vi "Example.vi"() -> ()   [LabVIEW 2018]
uses:
  <userlib>/DAQNavi Polymorphic VI/create/DAQNavi Create Channel(AI-Voltage).vi
  <userlib>/DAQNavi Polymorphic VI/configure/timing/DAQNavi Timing(AI Convert Clock).vi
  <userlib>/DAQNavi Polymorphic VI/read/DAQNavi Read (Analog 1D Wfm NChan NSamp).vi
  <userlib>/DAQNavi Polymorphic VI/configure/DAQNavi Get Property/Device/DAQNaviGet_Device_SupportedDevices_Ex.vi
  <vilib>/gmath/NI_Gmath.lvlib
panel:
  in  "MeanType":T1(ring)
  in  "Settings":T2(array[cluster])
  in  "Refresh Button":bool
  out "Acture Storage Period (s)":dbl=0.1 caption="Acture" min=0.001 format="%#_6p"
  out "Acture Refresh Period (s)":dbl=0.1 caption="Acture" min=0.001 format="%#_6p"
  in  "Storage Period (s)":dbl=0.1 min=0.001 format="%#_6p"
  out "File Path":path
  out "Recording":bool
  out "Over\nrun?":bool
  in  "Record Button":bool
  in  "Refresh Period (s)":dbl=0.1 min=0.001 format="%#_6p"
  in  "Process Stop Button":bool
  in  "Stop Button":bool
  in  "Play Button":bool
  out "Waveform Chart":waveform(dbl)[](graph)
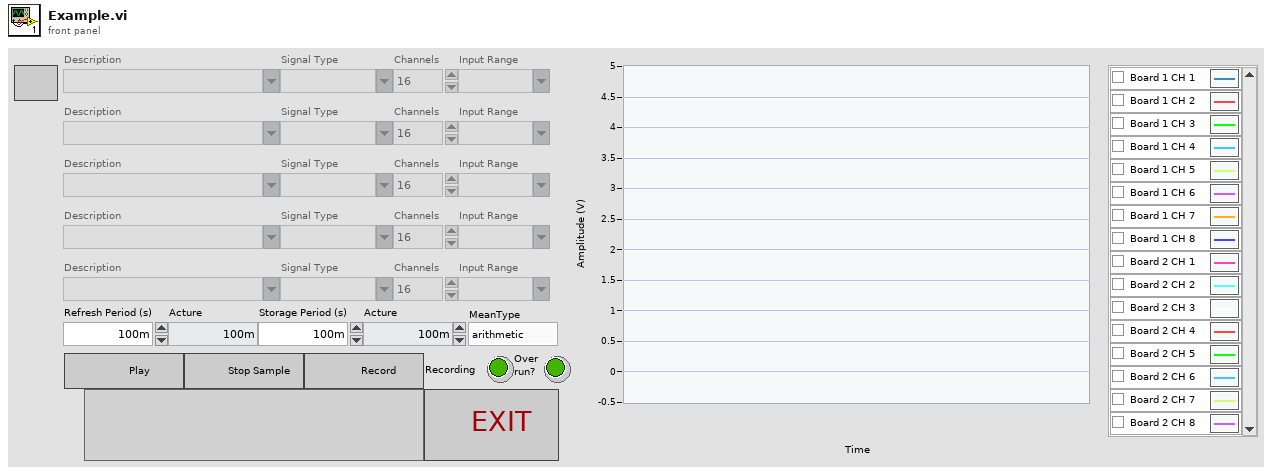
[diagram p1: front panel]
types:
  T1 = enum16{"arithmetic", "geometric", "harmonic", "trimmed", "median"}
  T2 = cluster{"Description":string, "Signal Type":string, "Channels":i32, "Input Range":string}[]
  T3 = enum16{"Close and Open", "Write", "Write Header", "Close"}
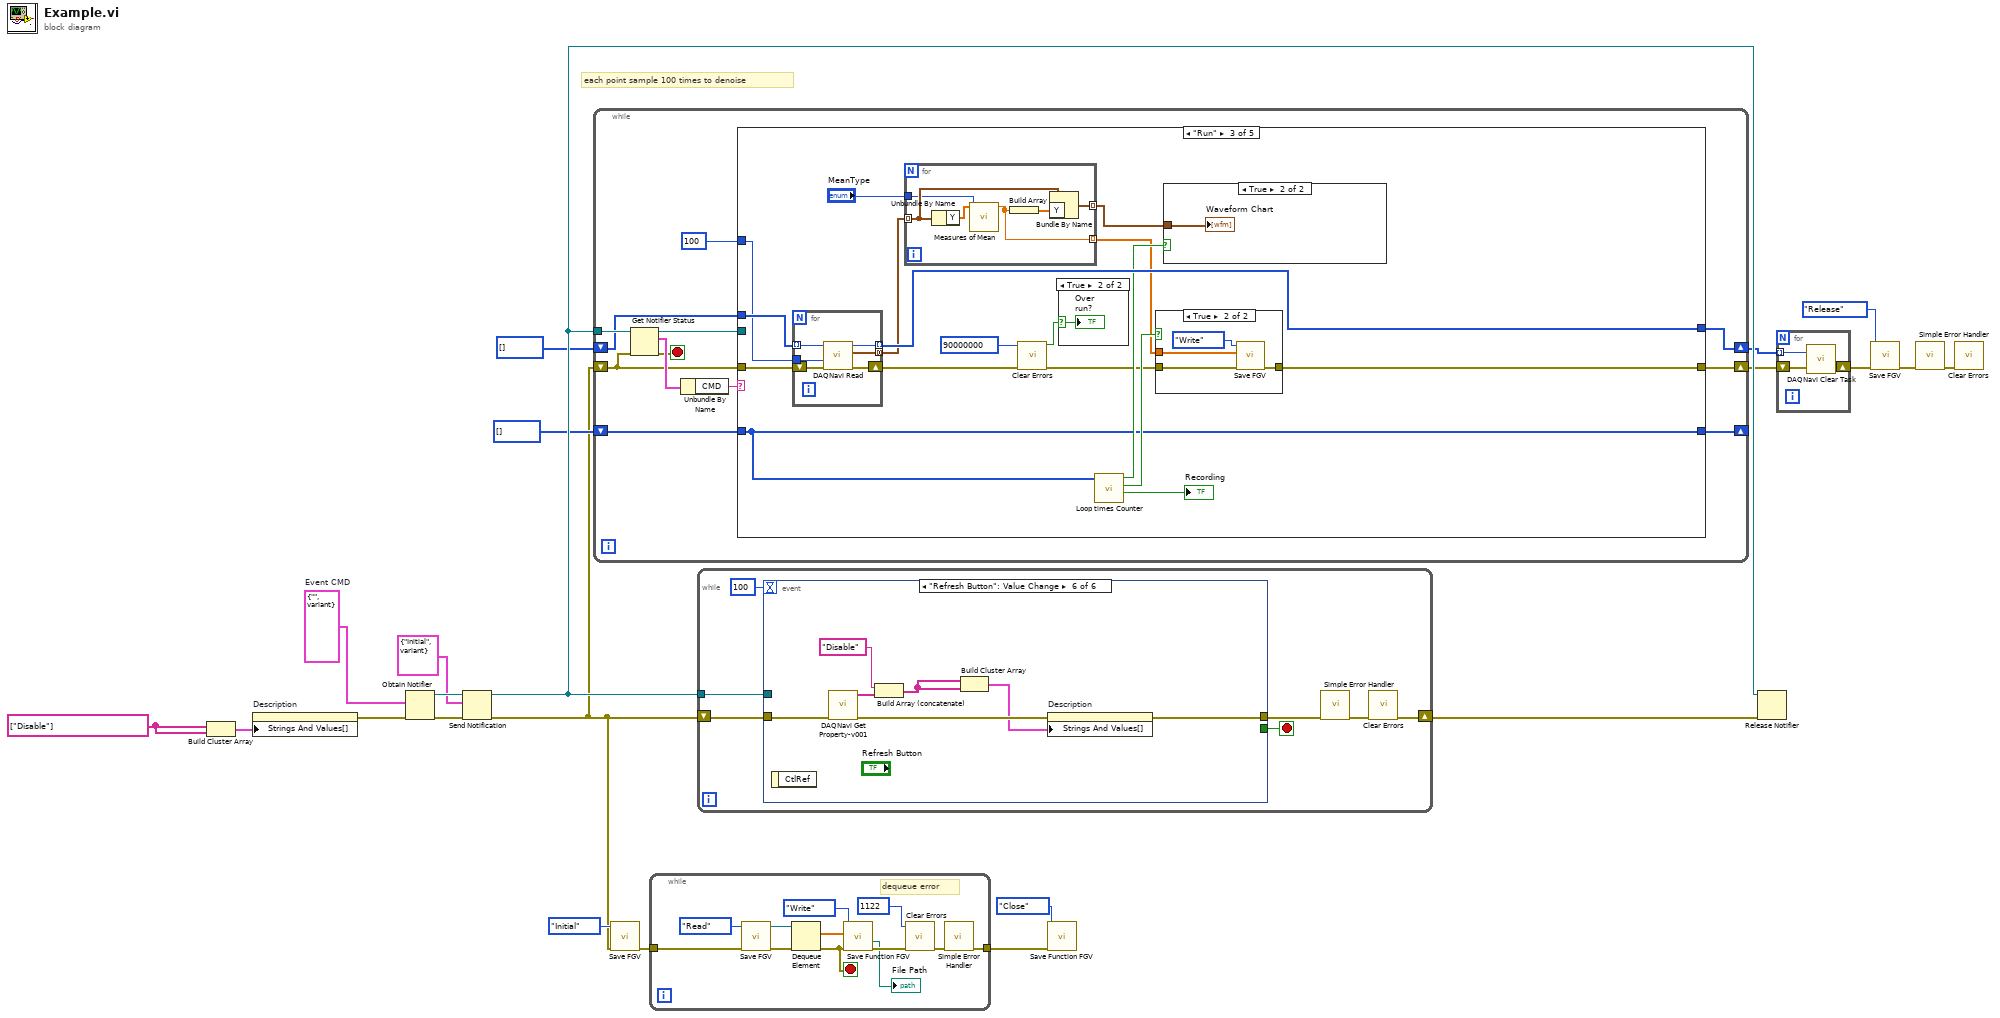
[diagram p0: block diagram]
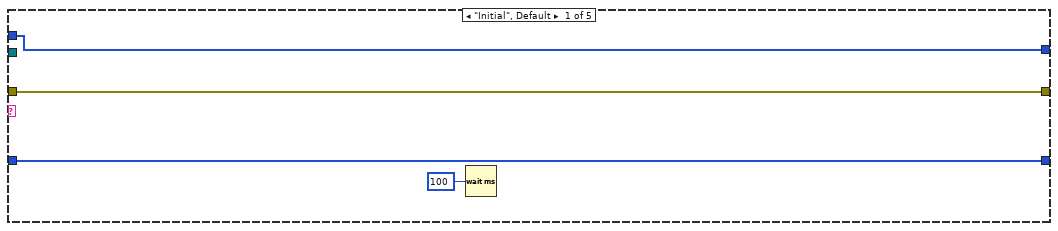
[diagram p2: hidden frame]
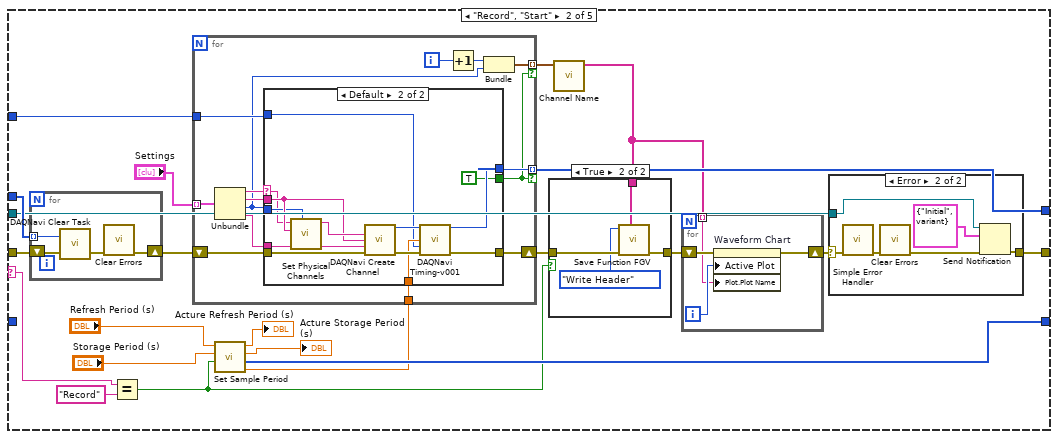
[diagram p3: hidden frame]
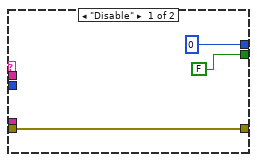
[diagram p5: hidden frame]
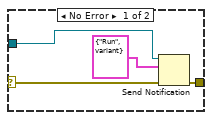
[diagram p6: hidden frame]
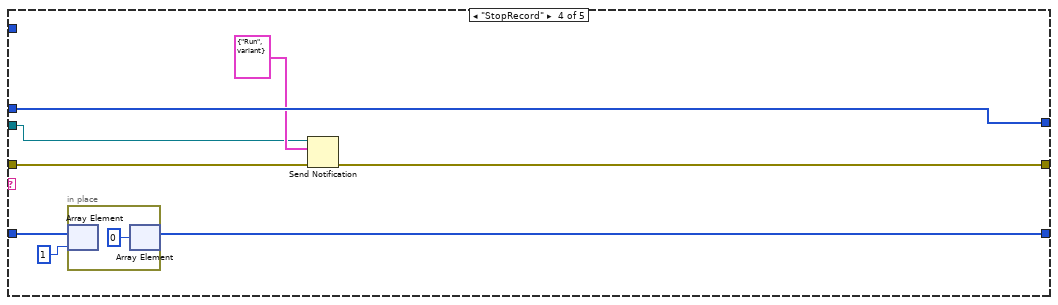
[diagram p10: hidden frame]
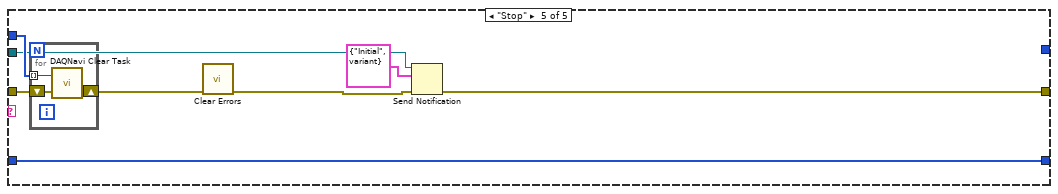
[diagram p11: hidden frame]
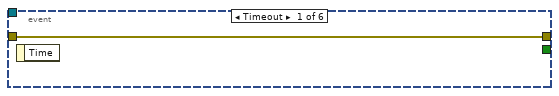
[diagram p12: hidden frame]
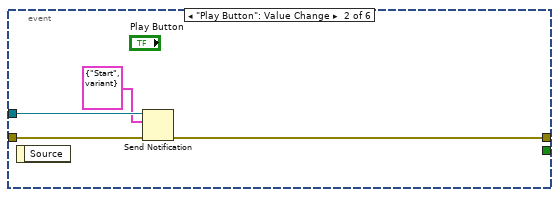
[diagram p13: hidden frame]
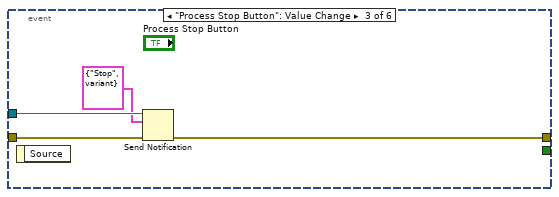
[diagram p14: hidden frame]
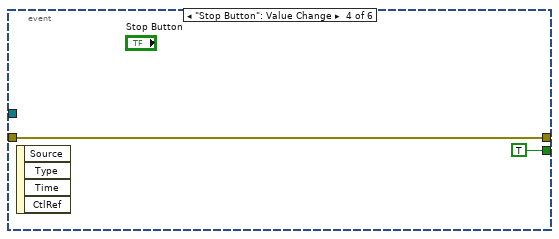
[diagram p15: hidden frame]
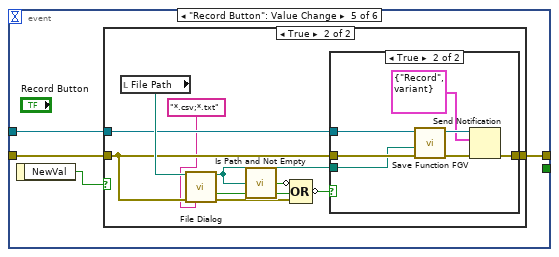
[diagram p16: hidden frame]
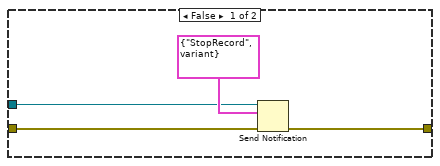
[diagram p17: hidden frame]
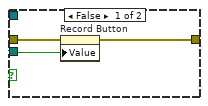
[diagram p18: hidden frame]
diagram:
  w3 = string[] ["Disable"]
  w22 = cluster{"CMD":string, "Data":variant} {"CMD"="", "Data"=variant}  # Event CMD
  # "each point sample 100 times to denoise"
  n1 = Build Cluster Array(w3, w3) -> (w2:cluster{"String":string, "String":string}[])
  n2 = property on="Description" class="CmbBox"("Strings And Values[]"=w2) -> (error out=w1:errorcluster)  [unwired: 2 in, 1 out]
  n3 = Obtain Notifier(notification data type=w22, error in (no error)=w1) -> (notifier out=w21:refnum<notifier>, error out=w19:errorcluster)  [unwired: 2 in, 1 out]
  n4 = Send Notification(notification=cluster{"CMD":string, "Data":variant} {"CMD"="Initial", "Data"=variant} ("element"), notifier=w21, error in (no error)=w19) -> (notifier out=w17:refnum<notifier>, error out=w10:errorcluster)
  n5 = while {
    tunnel: w17 -> [w34]
    shift-right: [w29] -> w7
    shift-left: i32[] [] ("task out") -> [w28]
    shift-right: [w24] -> w6
    shift-left: w10 -> [w30]
    shift-right: [w26] -> _
    shift-left: i32[] [] ("times") -> [w25]
    stop <- w31 stop-if-true
    n6 = Get Notifier Status(notifier=w34, error in (no error)=w30) -> (notifier out=w27:refnum<notifier>, current notification=w33:cluster{"CMD":string, "Data":variant}, error out=w31:errorcluster)  [unwired: 2 out]
    n7 = Unbundle By Name(w33) -> ("CMD"=w32:string)
    n8 = case shown="\"Run\"" w32 {
      selector: w32 -> [_ w45 _ _ _]
      tunnel: w30 -> [w38 w59 w125 w152 w164]
      tunnel: [w38 w51 w119 w151 w162] -> w24
      tunnel: [w37 w50 w129 w157 _] -> w29
      tunnel: w28 -> [w37 w60 w130 w157 w165]
      tunnel: w27 -> [_ w57 _ w150 w161]
      tunnel: [w35 w52 w122 w154 w159] -> w26
      tunnel: w25 -> [w35 _ w122 w156 w159]
      tunnel: u32 100 ("section length") -> [_ w48 w118 _ _]
      frame "Initial", Default {
        n9 = Wait (ms)(milliseconds to wait=u32 100) -> ()  [unwired: 1 out]
      }
      frame "Record", "Start" {
        n10 = for {
          tunnel: w60 -> [w73] mode=indexing
          shift-right: [w70] -> w58
          shift-left: w59 -> [w71]
          n11 = call <userlib>:"DAQNavi Clear Task.vi"("error in (no error)"=w71, "task in"=w73) -> ("error out"=w72:errorcluster)  [unwired: 1 out]
          n12 = call <vilib>:"Clear Errors.vi"("error in (no error)"=w72) -> ("error out"=w70:errorcluster)  [unwired: 5 in, 1 out]
        }
        n13 = Equal?(x=w45, y="Record") -> (x = y?=w43:bool)
        n14 = call "Set Sample Period.vi"("Record?"=w43, "Storage Period (s)"="Storage Period (s)", "Refresh Period (s)"="Refresh Period (s)") -> ("Rate"=w49:dbl, "times"=w52:i32[], "Acture Storage Period (s)"=→"Acture Storage Period (s)":dbl, "Acture Refresh Period (s)"=→"Acture Refresh Period (s)":dbl)  [unwired: 5 in]
        n15 = for {
          tunnel: [w85] -> w50 mode=indexing if=w74
          tunnel: w49 -> [w84]
          tunnel: w48 -> [w83]
          shift-right: [w86] -> w44
          shift-left: w58 -> [w87]
          tunnel: "Settings" -> [w82] mode=indexing
          tunnel: [w75] -> w42 mode=indexing if=w74
          i -> [w78]
          n16 = Unbundle(w82) -> ("Description"=w79:string, "Signal Type"=w81:string, "Channels"=w76:i32, "Input Range"=w80:string)
          n17 = case shown="Default" w79 {
            selector: w79 -> [_ w92]
            tunnel: w80 -> [_ w102]
            tunnel: w87 -> [w89 w101]
            tunnel: [w89 w98] -> w86
            tunnel: [0 ("task out") w97] -> w85
            tunnel: w84 -> [_ w96]
            tunnel: w83 -> [_ w95]
            tunnel: w81 -> [_ w94]
            tunnel: w76 -> [_ w93]
            tunnel: [FALSE TRUE] -> w74
            frame "Disable" {
            }
            frame Default {
              n18 = call "Set Physical Channels.vi"("Channels"=w93, "signal type"=w94, "Board Description"=w92) -> ("String"=w103:string)  [unwired: 8 in]
              n19 = call-poly <userlib>:"DAQNavi Create Channel.vi"("physical channels"=w103, "signal type"=w94, "value range"=w102, "error in (no error)"=w101) -> ("task out"=w100:i32, "error out"=w99:errorcluster)  [unwired: 1 in, 9 out]
              n20 = call-poly <userlib>:"DAQNavi Timing-v001.vi"("task in"=w100, "rate"=w96, "section length"=w95, "error in (no error)"=w99) -> ("task out"=w97:i32, "error out"=w98:errorcluster)  [unwired: 3 in, 7 out]
            }
          }
          n21 = Increment(x=w78) -> (x+1=w77:i32)
          n22 = Bundle(w77, "Channels"=w76) -> (w75:cluster{i32, "Channels":i32})  [unwired: 1 in]
        }
        n23 = call "Channel Name.vi"("Channel property"=w42) -> ("Channel Name"=w39:string[])  [unwired: 10 in]
        n24 = case shown="True" w43 {
          tunnel: w44 -> [w65 w69]
          tunnel: [w65 w68] -> w41
          tunnel: w39 -> [_ w67]
          frame False {
          }
          frame True {
            n25 = call "Save Function FGV.vi"("Channel Name in"=w67, "error in"=w69, "CMD"=T3."Write Header") -> ("error out"=w68:errorcluster)  [unwired: 6 in, 2 out]
          }
        }
        n26 = for {
          shift-right: [w63] -> w40
          shift-left: w41 -> [w64]
          tunnel: w39 -> [w61] mode=indexing
          i -> [w62]
          n27 = property on="Waveform Chart" class="WFChart (strict)"(error in=w64, "Active Plot"=w62, "Plot.Plot Name"=w61) -> (error out=w63:errorcluster)  [unwired: 1 in, 1 out]
        }
        n28 = case shown="Error" w40 {
          selector: w40 -> [w104 w110]
          tunnel: w57 -> [w107 w112]
          tunnel: [w106 w111] -> w51
          frame No Error {
            n29 = Send Notification(notification=cluster{"CMD":string, "Data":variant} {"CMD"="Run", "Data"=variant} ("element"), notifier=w107, error in (no error)=w104) -> (error out=w106:errorcluster)  [unwired: 1 out]
          }
          frame Error {
            n30 = call <vilib>:"Simple Error Handler.vi"("error in (no error)"=w110) -> ("error out"=w109:errorcluster)  [unwired: 4 in, 4 out]
            n31 = call <vilib>:"Clear Errors.vi"("error in (no error)"=w109) -> ("error out"=w108:errorcluster)  [unwired: 5 in, 1 out]
            n32 = Send Notification(notification=cluster{"CMD":string, "Data":variant} {"CMD"="Initial", "Data"=variant} ("element"), notifier=w112, error in (no error)=w108) -> (error out=w111:errorcluster)  [unwired: 1 out]
          }
        }
      }
      frame "Run" {
        n33 = for {
          tunnel: w130 -> [w136] mode=indexing
          tunnel: [w135] -> w129 mode=indexing
          tunnel: w118 -> [w132]
          tunnel: [w131] -> w116 mode=concatenating
          shift-right: [w134] -> w128
          shift-left: w125 -> [w133]
          n34 = call-poly <userlib>:"DAQNavi Read.vi"("error in (no error)"=w133, "number of samples per channel to read"=w132, "task in"=w136) -> ("error out"=w134:errorcluster, "data"=w131:waveform(dbl)[], "task out"=w135:i32)  [unwired: 1 in, 5 out]
        }
        n35 = for {
          tunnel: w116 -> [w145] mode=indexing
          tunnel: [w146] -> w115 mode=indexing
          tunnel: [w148] -> w117 mode=indexing
          tunnel: "MeanType" -> [w144]
          n36 = Unbundle By Name(w145) -> ("Y"=w149:dbl[])
          n37 = call <vilib>:"Measures of Mean.vi"("type"=w144, "x array"=w149) -> ("mean value"=w148:dbl)  [unwired: 8 in, 1 out]
          n38 = Build Array(w148) -> (w147:dbl[])
          n39 = Bundle By Name(cluster=w145, "Y"=w147) -> (w146:waveform(dbl))
        }
        n40 = call <vilib>:"Clear Errors.vi"("error in (no error)"=w128, "specific error code to clear (0: all)"=90000000) -> ("error out"=w120:errorcluster, "specific error cleared?"=w126:bool)  [unwired: 4 in]
        n41 = case shown="True" w126 {
          selector: w126 -> [_ w143]
          frame False {
          }
          frame True {
            "Over\nrun?" <- w143
          }
        }
        n42 = call "Loop times Counter.vi"("times"=w122) -> ("Recording?"=→"Recording":bool, "Save file?"=w123:bool, "Display value?"=w124:bool)  [unwired: 8 in]
        n43 = case shown="True" w123 {
          tunnel: w117 -> [_ w141]
          tunnel: w120 -> [w137 w140]
          tunnel: [w137 w138] -> w119
          frame False {
          }
          frame True {
            n44 = call "Save FGV.vi"("error in (no error)"=w140, "Data in"=w141, "CMD"=enum16{"Initial", "Read", "Write", "Release"}."Write") -> ("error out"=w138:errorcluster)  [unwired: 7 in, 1 out]
          }
        }
        n45 = case shown="True" w124 {
          tunnel: w115 -> [_ w142]
          frame False {
          }
          frame True {
            "Waveform Chart" <- w142
          }
        }
      }
      frame "StopRecord" {
        n46 = in-place {
          n47 = in-place-array #1(w156, 1) -> ()  [unwired: 1 out]
          n48 = in-place-array #1(0 ("element")) -> (w154:i32[])  [unwired: 1 out]
        }
        n49 = Send Notification(notification=cluster{"CMD":string, "Data":variant} {"CMD"="Run", "Data"=variant} ("element"), notifier=w150, error in (no error)=w152) -> (error out=w151:errorcluster)  [unwired: 1 out]
      }
      frame "Stop" {
        n50 = for {
          tunnel: w165 -> [w168] mode=indexing
          shift-right: [w169] -> w166
          shift-left: w164 -> [w167]
          n51 = call <userlib>:"DAQNavi Clear Task.vi"("error in (no error)"=w167, "task in"=w168) -> ("error out"=w169:errorcluster)  [unwired: 1 out]
        }
        n52 = call <vilib>:"Clear Errors.vi"("error in (no error)"=w166) -> ("error out"=w163:errorcluster)  [unwired: 5 in, 1 out]
        n53 = Send Notification(notification=cluster{"CMD":string, "Data":variant} {"CMD"="Initial", "Data"=variant} ("element"), notifier=w161, error in (no error)=w163) -> (error out=w162:errorcluster)  [unwired: 1 out]
      }
    }
  }
  n54 = call "Save FGV.vi"("error in (no error)"=w10, "CMD"=enum16{"Initial", "Read", "Write", "Release"}."Initial") -> ("error out"=w12:errorcluster)  [unwired: 8 in, 1 out]
  n55 = while {
    tunnel: w12 -> [w180]
    tunnel: [w173] -> w11
    stop <- w176 stop-if-true
    # "dequeue error"
    n56 = call "Save FGV.vi"("error in (no error)"=w180, "CMD"=enum16{"Initial", "Read", "Write", "Release"}."Read") -> ("error out"=w177:errorcluster, "file queue out"=w179:refnum<queue>)  [unwired: 8 in]
    n57 = Dequeue Element(queue=w179, error in (no error)=w177) -> (element=w178:dbl[], error out=w176:errorcluster)  [unwired: 1 in, 2 out]
    n58 = call "Save Function FGV.vi"("error in"=w176, "data in"=w178, "CMD"=T3."Write") -> ("error out"=w175:errorcluster, "file path out"=→"File Path":path)  [unwired: 6 in, 1 out]
    n59 = call <vilib>:"Clear Errors.vi"("error in (no error)"=w175, "specific error code to clear (0: all)"=1122) -> ("error out"=w174:errorcluster)  [unwired: 4 in, 1 out]
    n60 = call <vilib>:"Simple Error Handler.vi"("error in (no error)"=w174) -> ("error out"=w173:errorcluster)  [unwired: 4 in, 4 out]
  }
  n61 = while {
    tunnel: w17 -> [w188]
    shift-right: [w183] -> w18
    shift-left: w10 -> [w185]
    stop <- w186 stop-if-true
    n62 = event shown="[5] \"Refresh Button\": Value Change" {
      selector: _ -> [_ _ _ _ _ _]
      dyn-events: _ -> [_ _ _ _ _ _]
      timeout: 100 -> [_ _ _ _ _ _]
      tunnel: w188 -> [_ w193 w197 _ w201 _]
      tunnel: [w189 w192 w196 w198 w202 w229] -> w187
      tunnel: [_ _ _ TRUE _ _] -> w186
      tunnel: w185 -> [w189 w190 w194 w198 w203 w233]
      event Timeout {
        n63 = event-data() -> ()  [unwired: 1 in, 1 out]
      }
      event "Play Button": Value Change {
        n64 = event-data() -> ()  [unwired: 1 in, 1 out]
        n65 = Send Notification(notification=cluster{"CMD":string, "Data":variant} {"CMD"="Start", "Data"=variant} ("element"), notifier=w193, error in (no error)=w190) -> (error out=w192:errorcluster)  [unwired: 1 out]
      }
      event "Process Stop Button": Value Change {
        n66 = event-data() -> ()  [unwired: 1 in, 1 out]
        n67 = Send Notification(notification=cluster{"CMD":string, "Data":variant} {"CMD"="Stop", "Data"=variant} ("element"), notifier=w197, error in (no error)=w194) -> (error out=w196:errorcluster)  [unwired: 1 out]
      }
      event "Stop Button": Value Change {
        n68 = event-data() -> ()  [unwired: 1 in, 4 out]
      }
      event "Record Button": Value Change {
        n69 = event-data() -> ("NewVal"=w200:bool)  [unwired: 1 in]
        n70 = case shown="True" w200 {
          tunnel: w203 -> [w205 w211]
          tunnel: [w204 w210] -> w202
          tunnel: w201 -> [w206 w209]
          frame False {
            n71 = Send Notification(notification=cluster{"CMD":string, "Data":variant} {"CMD"="StopRecord", "Data"=variant} ("element"), notifier=w206, error in (no error)=w205) -> (error out=w204:errorcluster)  [unwired: 1 out]
          }
          frame True {
            n72 = local read "File Path"() -> (w212:path)
            n73 = call "File Dialog"("start path"=w212, "error in"=w211, "pattern (all files)"="*.csv;*.txt") -> ("selected path"=w214:path, "cancelled"=w216:bool, "error out"=w215:errorcluster)  [unwired: 9 in, 1 out]
            n74 = call <vilib>:"Is Path and Not Empty.vi"("path"=w214) -> ("Is Path and Not Empty?"=w217:bool)  [unwired: 4 in]
            n75 = Compound Arithmetic op=OR(invert w217, w216, w215) -> (invert w213:bool)
            n76 = case shown="True" w213 {
              selector: w213 -> [w218 _]
              tunnel: w214 -> [_ w221]
              tunnel: w211 -> [w220 w223]
              tunnel: [w219 w226] -> w210
              tunnel: w209 -> [_ w225]
              frame False {
                n77 = property on="Record Button" class="Bool (strict)"(error in=w220, "Value"=w218) -> (error out=w219:errorcluster)  [unwired: 1 in, 1 out]
              }
              frame True {
                n78 = call "Save Function FGV.vi"("error in"=w223, "file path in"=w221) -> ("error out"=w222:errorcluster)  [unwired: 7 in, 2 out]
                n79 = Send Notification(notification=cluster{"CMD":string, "Data":variant} {"CMD"="Record", "Data"=variant} ("element"), notifier=w225, error in (no error)=w222) -> (error out=w226:errorcluster)  [unwired: 1 out]
              }
            }
          }
        }
      }
      event "Refresh Button": Value Change {
        n80 = event-data() -> ()  [unwired: 1 in, 1 out]
        n81 = call-poly <userlib>:"DAQNavi Get Property-v001.vi"("error in (no error)"=w233) -> ("error out"=w231:errorcluster, "supported devices"=w232:string[])  [unwired: 9 in]
        n82 = Build Array (concatenate)("Disable", w232) -> (w228:string[])
        n83 = Build Cluster Array(w228, w228) -> (w230:cluster{"String":string, "String":string}[])
        n84 = property on="Description" class="CmbBox"(error in=w231, "Strings And Values[]"=w230) -> (error out=w229:errorcluster)  [unwired: 1 in, 1 out]
      }
    }
    n85 = call <vilib>:"Simple Error Handler.vi"("error in (no error)"=w187) -> ("error out"=w184:errorcluster)  [unwired: 4 in, 4 out]
    n86 = call <vilib>:"Clear Errors.vi"("error in (no error)"=w184) -> ("error out"=w183:errorcluster)  [unwired: 5 in, 1 out]
  }
  n87 = call "Save Function FGV.vi"("error in"=w11, "CMD"=T3."Close") -> ()  [unwired: 7 in, 3 out]
  n88 = Release Notifier(notifier=w17, error in (no error)=w18) -> ()  [unwired: 1 in, 3 out]
  n89 = for {
    tunnel: w7 -> [w236] mode=indexing
    shift-right: [w234] -> w5
    shift-left: w6 -> [w235]
    n90 = call <userlib>:"DAQNavi Clear Task.vi"("error in (no error)"=w235, "task in"=w236) -> ("error out"=w234:errorcluster)  [unwired: 1 out]
  }
  n91 = call "Save FGV.vi"("error in (no error)"=w5, "CMD"=enum16{"Initial", "Read", "Write", "Release"}."Release") -> ("error out"=w8:errorcluster)  [unwired: 8 in, 1 out]
  n92 = call <vilib>:"Simple Error Handler.vi"("error in (no error)"=w8) -> ("error out"=w9:errorcluster)  [unwired: 4 in, 4 out]
  n93 = call <vilib>:"Clear Errors.vi"("error in (no error)"=w9) -> ()  [unwired: 5 in, 2 out]
